vi "poly_now_ms_timer.vi"(8 "Error in":errorcluster caption="Error in (no error)") -> (0 "Error out":errorcluster, 2 "millisecond timer value":i32)   [LabVIEW 2015]
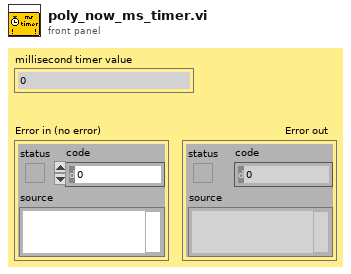
[diagram p1: front panel]
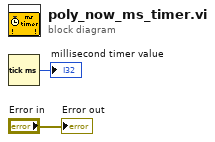
[diagram p0: block diagram]
diagram:
  n1 = Tick Count (ms)() -> (millisecond timer value=→"millisecond timer value":u32)
  "Error out" <- "Error in"
